vi "Switch Configuration.vi"(6 "Write? (f)":bool, 7 "Connection Refnum":T2, 8 "error in (no error)":errorcluster, 9 "Configuration (\"\")":string, 11 "Template Keys (empty)":T1) -> (0 "error out":errorcluster, 1 "Configuration":string, 3 "Template Keys":T1, 5 "Connection Refnum":T2)   [LabVIEW 2011]
uses:
  Summitek EXT/ODBC/SQL Controls/Connection Refnum.ctl
  ITK EXT/utils/keyedarr.llb/Keyed Array.ctl
  ITK EXT/utils/strutil.llb/Case Matching.ctl
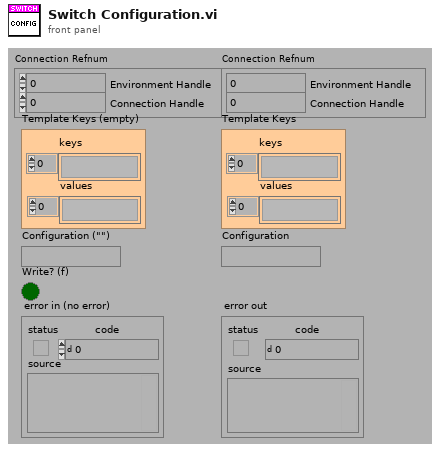
[diagram p1: front panel]
types:
  T1 = typedef "Keyed Array.ctl" = cluster{"keys":string[], "values":string[]}
  T2 = typedef "Connection Refnum.ctl" = cluster{"Environment Handle":i32, "Connection Handle":i32}
  T3 = typedef "Case Matching.ctl" = enum16{"a != A", "a == A", "system"}
  T4 = typedef "Switch Test Parameters.ctl" = cluster{"Stimulus":T5, "Switch Info":T7}
  T5 = typedef "Switch Stimulus Parameters.ctl" = cluster{"Blank Screen":bool, "SWI Position":variant, "Switch Type":T6}
  T6 = typedef "Switch Type.ctl" = enum16{"Sea-Level", "Simulator", "SI-0206-SW", "SI-0309-SW", "SI-0310-SW", "Front End"}
  T7 = typedef "Switch Instrument Info.ctl" = cluster{"sDriverId":string, "sDriverType":string, "Model":string, "Serial":string, "USB Serial":string}
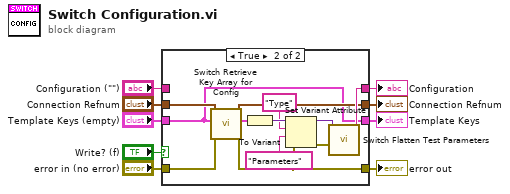
[diagram p0: block diagram]
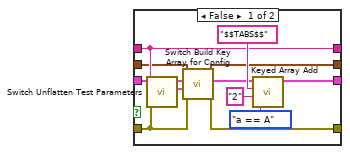
[diagram p2: hidden frame]
diagram:
  n1 = case shown="True" "Write? (f)" {
    tunnel: "error in (no error)" -> [w10 w27]
    tunnel: [w14 w22] -> w8
    tunnel: "Template Keys (empty)" -> [w12 w22]
    tunnel: "Configuration (\"\")" -> [w18 _]
    tunnel: [w13 w26] -> w5
    tunnel: [w18 w28] -> w4
    tunnel: "Connection Refnum" -> [w17 w25]
    tunnel: [w16 w24] -> w1
    frame False {
      n2 = call "Switch Unflatten Test Parameters.vi"("error in (no error)"=w10, "Parameter String"=w18) -> ("Switch Test Parameters"=w11:T4)  [unwired: 9 out]
      n3 = call "Switch Build Key Array for Config.vi"("error in (no error)"=w10, "Switch Test Parameters"=w11, "Key Array In"=w12, "Connection Refnum"=w17) -> ("error out"=w13:errorcluster, "Key Array Out"=w15:T1, "Connection Refnum"=w16:T2)  [unwired: 5 out]
      n4 = call "Keyed Array Add.vi"("case matching (sensitive)"=Case_Matching."a == A", "value"="2", "key"="$$TABS$$", "array in"=w15) -> ("array out"=w14:T1)  [unwired: 3 out]
    }
    frame True {
      n5 = call "Switch Retrieve Key Array for Config.vi"("error in (no error)"=w27, "Key Array In"=w22, "Connection Refnum"=w25) -> ("error out"=w26:errorcluster, "Switch Test Parameters"=w23:T4, "Connection Refnum"=w24:T2)  [unwired: 1 in, 5 out]
      n6 = To Variant(anything=w23) -> (Variant=w33:variant)
      n7 = Set Variant Attribute(Variant=w33, name="Type", value="Parameters" ("name"), error in=w26) -> (Variant out=w29:variant, error out=w32:errorcluster)  [unwired: 1 out]
      n8 = call "Switch Flatten Test Parameters.vi"("error in (no error)"=w32, "Parameter Variant"=w29) -> ("Parameter String"=w28:string)  [unwired: 9 out]
    }
  }
  "error out" <- w5
  "Connection Refnum" <- w1
  "Template Keys" <- w8
  "Configuration" <- w4
